vi "HW_Gantner_Init Port.vi"(8 "错误输入":errorcluster caption="错误输入（无错误）", 11 "IPAddress":string) -> (0 "错误输出":errorcluster)   [LabVIEW 2016]
uses:
  ISMBUS32.DLL
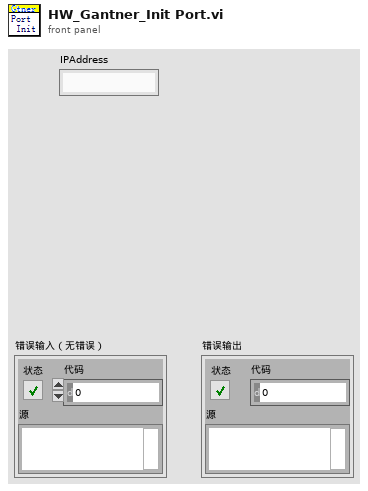
[diagram p1: front panel]
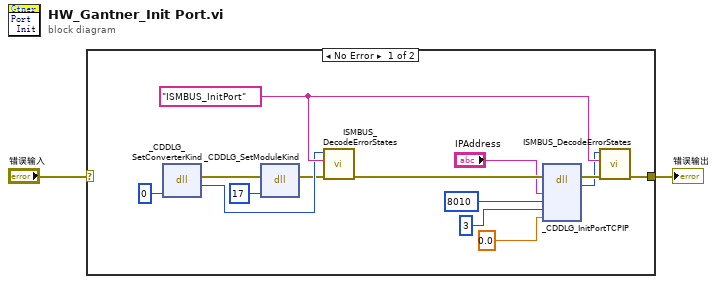
[diagram p0: block diagram]
diagram:
  n1 = case shown="No Error" "错误输入" {
    selector: "错误输入" -> [_ w17]
    tunnel: [w16 w17] -> w2
    frame No Error {
      w15 = "ISMBUS_InitPort" ("Location")
      n2 = dll-call lib="Ismbus32.dll" fn="_CDDLG_SetConverterKind"("ConverterKind"=0) -> (error out=w11:errorcluster, "Rückgabetyp"=w13:i32)  [unwired: 4 in, 1 out]
      n3 = dll-call lib="Ismbus32.dll" fn="_CDDLG_SetModuleKind"(error in=w11, "Modulekind"=17) -> (error out=w12:errorcluster)  [unwired: 3 in, 2 out]
      n4 = call "ISMBUS_DecodeErrorStates.vi"("Fehler (Eingang - kein Fehler)"=w12, "Location"=w15, "ISMBUS_Error State"=w13) -> ("Fehler (Ausgang)"=w9:errorcluster)  [unwired: 8 out]
      n5 = dll-call lib="Ismbus32.dll" fn="_CDDLG_InitPortTCPIP"(error in=w9, "IPAddr"="IPAddress", "IPPort"=8010, "Prot"=3, "TimeoutS"=0.0) -> (error out=w5:errorcluster, "Rückgabetyp"=w4:i32)  [unwired: 6 in, 1 out]
      n6 = call "ISMBUS_DecodeErrorStates.vi"("Fehler (Eingang - kein Fehler)"=w5, "Location"=w15, "ISMBUS_Error State"=w4) -> ("Fehler (Ausgang)"=w16:errorcluster)  [unwired: 8 out]
    }
    frame Error {
    }
  }
  "错误输出" <- w2
